vi "Test PJVS.vi"(8 "error in (pass through)":errorcluster, 11 "PJVS setup":T1={"PJVS type"=enum."AC-supraVOLTcontrol", "Status Refnum"=refnum, "AC-supraVOLTcontrol"={"IP address:port (0.0.0.0:0000)"="0.0.0.0:0000", "Timeouts"={"TCP Read & Write (ms)"=7000, "Sensors readout"=5000, "PJVS setup"=10000, "Nullmeter readout"=5000, "Multiplexer setup"=3000, "57XX setup"=15000, "Generator setup"=5000, "Synthesizer setup"=3000, "Sampler readout"=10000}, "Simulation mode"=FALSE, "Debug mode"=FALSE}, "NPL bias source"={"DataSocketCluster"={"Server Machine"="CZC", "Client Machine"="localhost", "Data"="P2", "TimeStamp"=0.0, "Count"=1, "Target Process"="General Server"}}, "Manual PJVS"={"PJVS frequency (Hz)"=0.0, "Reference voltages (V)"=[], "File with PJVS voltages"=path ""}, "VTT PJVS"={"some VTT only property"=""}} {"NPL bias source"."DataSocketCluster"."TimeStamp" format="%.2f"}) -> (0 "error out":errorcluster, 2 "Status":string, 3 "PJVS setup out":T1={"PJVS type"=enum."AC-supraVOLTcontrol", "Status Refnum"=refnum, "AC-supraVOLTcontrol"={"IP address:port (0.0.0.0:0000)"="0.0.0.0:0000", "Timeouts"={"TCP Read & Write (ms)"=7000, "Sensors readout"=5000, "PJVS setup"=10000, "Nullmeter readout"=5000, "Multiplexer setup"=3000, "57XX setup"=15000, "Generator setup"=5000, "Synthesizer setup"=3000, "Sampler readout"=10000}, "Simulation mode"=FALSE, "Debug mode"=FALSE}, "NPL bias source"={"DataSocketCluster"={"Server Machine"="CZC", "Client Machine"="localhost", "Data"="P2", "TimeStamp"=0.0, "Count"=1, "Target Process"="General Server"}}, "Manual PJVS"={"PJVS frequency (Hz)"=0.0, "Reference voltages (V)"=[], "File with PJVS voltages"=path ""}, "VTT PJVS"={"some VTT only property"=""}} {"NPL bias source"."DataSocketCluster"."TimeStamp" format="%.2f"})   [LabVIEW 2020]
doc: "Tests communication with PJVS system."
uses:
  Type definitions/PJVS.ctl
  Type definitions/PJVS Type.ctl
  external libraries/acsvcontrol-driver/Public/Type Definitions/Timeouts.ctl
  external libraries/JV modified NPL Bias source/DataSocketCluster external.ctl
  <vilib>/Utility/error.llb/DialogType.ctl
  external libraries/acsvcontrol-driver/ACSVcontrol-driver.lvlib
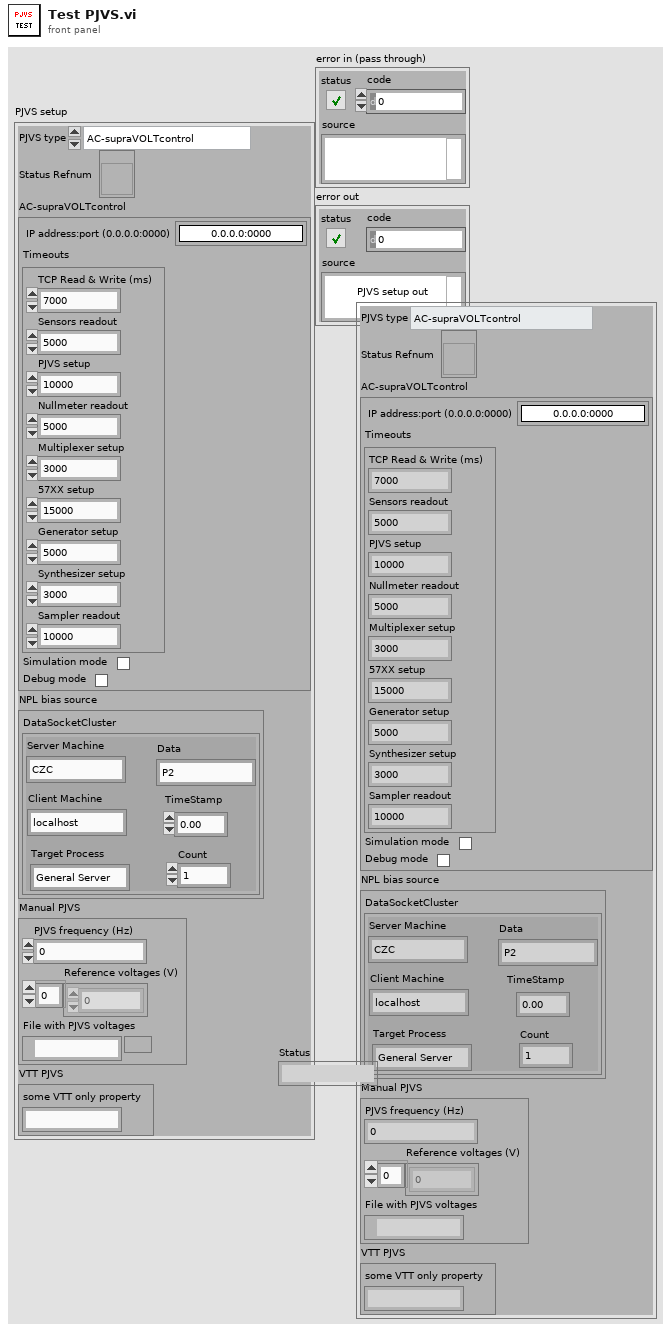
[diagram p1: front panel]
types:
  T1 = typedef "PJVS.ctl" = cluster{"PJVS type":T2, "Status Refnum":refnum<vi>, "AC-supraVOLTcontrol":cluster{"IP address:port (0.0.0.0:0000)":string, "Timeouts":T3, "Simulation mode":bool, "Debug mode":bool}, "NPL bias source":cluster{"DataSocketCluster":T4}, "Manual PJVS":cluster{"PJVS frequency (Hz)":dbl, "Reference voltages (V)":dbl[], "File with PJVS voltages":path}, "VTT PJVS":cluster{"some VTT only property":string}}
  T2 = typedef "PJVS Type.ctl" = enum16{"AC-supraVOLTcontrol", "JV modified NPL bias control", "Manual PJVS", "VTT PJVS"}
  T3 = typedef "ACSVcontrol-driver.lvlib/Timeouts.ctl" = cluster{"TCP Read & Write (ms)":i32, "Sensors readout":i32, "PJVS setup":i32, "Nullmeter readout":i32, "Multiplexer setup":i32, "57XX setup":i32, "Generator setup":i32, "Synthesizer setup":i32, "Sampler readout":i32}
  T4 = typedef "DataSocketCluster external.ctl" = cluster{"Server Machine":string, "Client Machine":string, "Data":string, "TimeStamp":dbl, "Count":i32, "Target Process":string}
  T5 = typedef "DialogType.ctl" = u16
  T6 = typedef "ACSVcontrol-driver.lvlib/Sensors Data.ctl" = cluster{"Temperature (°C)":dbl, "Barometric Pressure (mbar)":dbl, "Humidity (%)":dbl, "Temperature Cooler (K)":dbl}
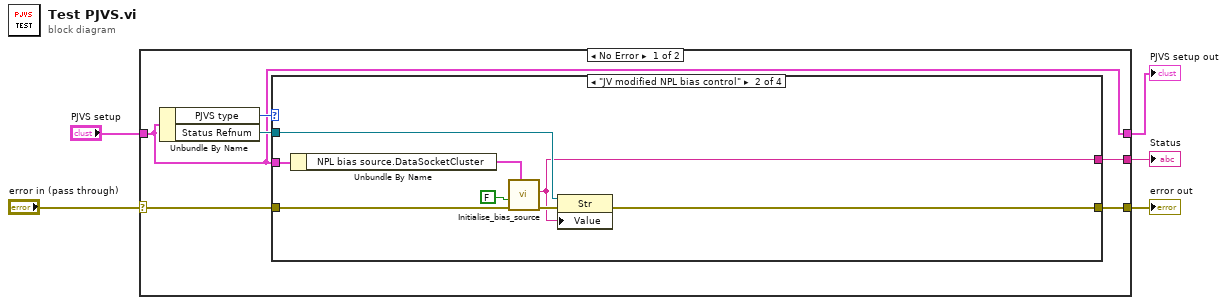
[diagram p0: block diagram]
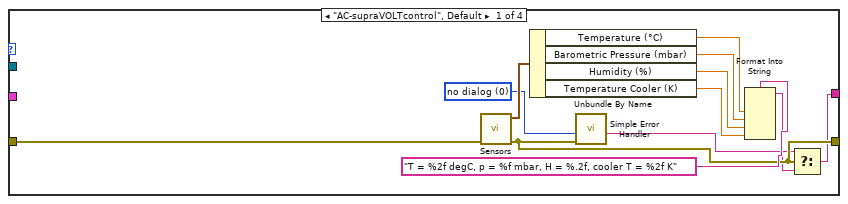
[diagram p2: hidden frame]
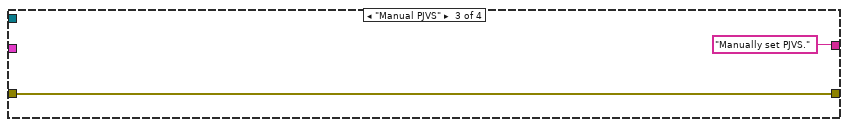
[diagram p3: hidden frame]
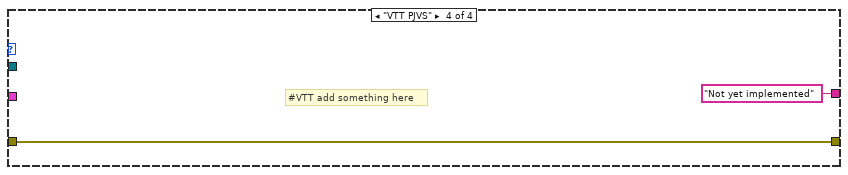
[diagram p4: hidden frame]
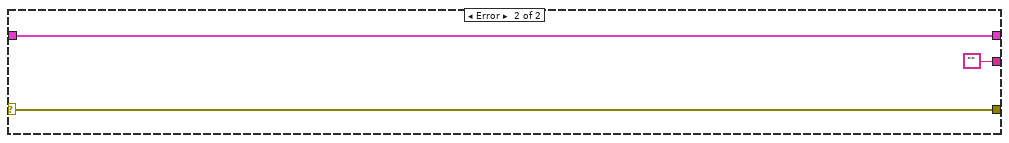
[diagram p5: hidden frame]
diagram:
  n1 = case shown="No Error" "error in (pass through)" {
    selector: "error in (pass through)" -> [w8 w38]
    tunnel: "PJVS setup" -> [w6 w37]
    tunnel: [w9 w38] -> w4
    tunnel: [w6 w37] -> w2
    tunnel: [w7 ""] -> w1
    frame No Error {
      n2 = Unbundle By Name(w6) -> ("PJVS type"=w11:T2, "Status Refnum"=w10:refnum<vi>)
      n3 = case shown="\"JV modified NPL bias control\"" w11 {
        tunnel: w10 -> [_ w27 _ _]
        tunnel: w8 -> [w23 w30 w32 w35]
        tunnel: [w15 w25 w32 w35] -> w9
        tunnel: [w12 w24 "Manually set PJVS." ("Response Initialise") "Not yet implemented" ("Response Initialise")] -> w7
        tunnel: w6 -> [_ w29 _ _]
        frame "AC-supraVOLTcontrol", Default {
          w16 = T5 0 items=["no dialog", "OK message", "continue or stop message", "OK message + warnings", "continue/stop + warnings"] ("type of dialog (OK msg:1)")
          n4 = call "Sensors.vi"("error in (no error)"=w23) -> ("error out"=w15:errorcluster, "Sensors Data"=w21:T6)  [unwired: 9 in]
          n5 = Unbundle By Name(w21) -> ("Temperature (°C)"=w20:dbl, "Barometric Pressure (mbar)"=w19:dbl, "Humidity (%)"=w18:dbl, "Temperature Cooler (K)"=w17:dbl)
          n6 = call <vilib>:"Simple Error Handler.vi"("type of dialog (OK msg:1)"=w16, "error in (no error)"=w15) -> ("source out"=w14:string)  [unwired: 3 in, 4 out]
          n7 = Format Into String(format string="T = %2f degC, p = %f mbar, H = %.2f, cooler T = %2f K", w20, w19, w18, w17) -> (resulting string=w13:string)  [unwired: 2 in, 1 out]
          n8 = Select(t=w14, s=w15, f=w13) -> (s? t:f=w12:string)
        }
        frame "JV modified NPL bias control" {
          n9 = Unbundle By Name(w29) -> ("NPL bias source.DataSocketCluster"=w28:T4)
          n10 = call "Initialise_bias_source.vi"("output cluster"=w28, "error in (no error)"=w30, "Load bias parameters"=FALSE) -> ("error out"=w26:errorcluster, "Response Initialise"=w24:string)  [unwired: 6 in, 1 out]
          n11 = property class="Str"(reference=w27, error in=w26, "Value"=w24) -> (error out=w25:errorcluster)  [unwired: 1 out]
        }
        frame "Manual PJVS" {
        }
        frame "VTT PJVS" {
          # "#VTT add something here"
        }
      }
    }
    frame Error {
    }
  }
  "error out" <- w4
  "PJVS setup out" <- w2
  "Status" <- w1
